vi "LASERs_ Crl_AE.vi"(7 "Action":enum16{"READ", "WRITE"}(ring), 10 "Laser Parameters In":T1 {"405 Power (0-5V)" min=0.0 max=5.0}) -> (2 "Laser Parameters Out":T1 {"405 Power (0-5V)" min=0.0 max=5.0})   [LabVIEW 2016]
uses:
  Host VIs/Laser Controls.ctl
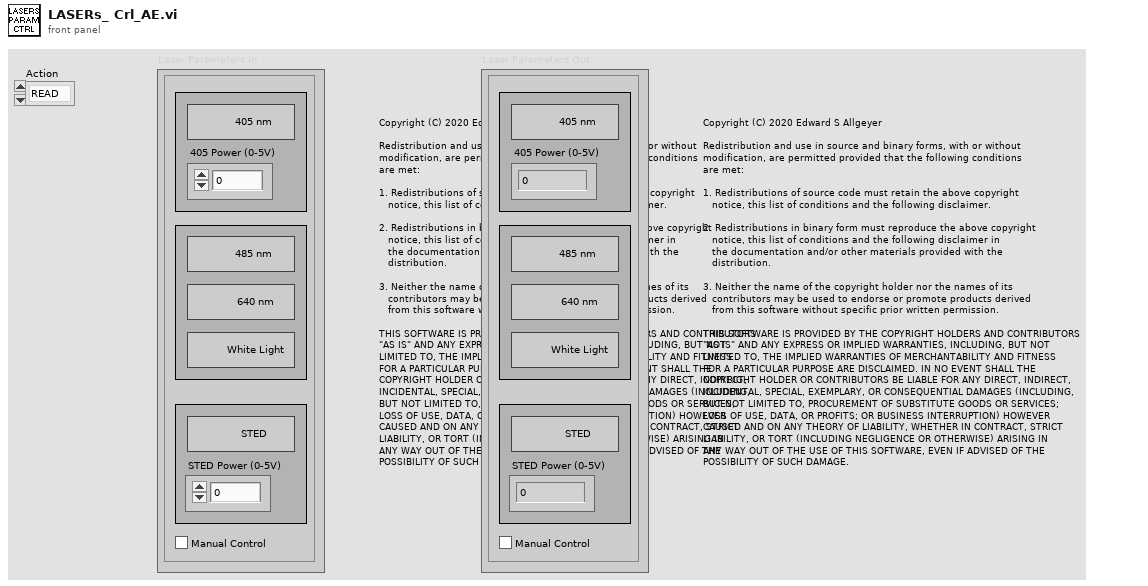
[diagram p1: front panel]
types:
  T1 = typedef "Laser Controls.ctl" = cluster{"STED Power (0-5V)":dbl, "STED":bool, "640 nm":bool, "485 nm":bool, "Manual Control":bool, "White Light":bool, "405 nm":bool, "405 Power (0-5V)":dbl}
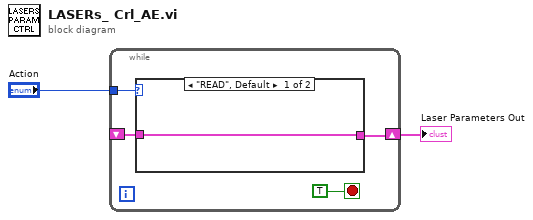
[diagram p0: block diagram]
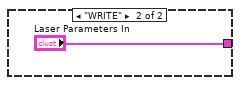
[diagram p2: hidden frame]
diagram:
  n1 = while {
    tunnel: "Action" -> [w5]
    shift-right: [w4] -> w1
    shift-left: _ -> [w3]
    stop <- TRUE stop-if-true
    n2 = case shown="\"READ\", Default" w5 {
      tunnel: [w7 "Laser Parameters In"] -> w4
      tunnel: w3 -> [w7 _]
      frame "READ", Default {
      }
      frame "WRITE" {
      }
    }
  }
  "Laser Parameters Out" <- w1
